vi "Read Access Key.vi"(8 "error in (no error)":errorcluster, 11 "HTTP Session in":refnum<class "Session.lvclass">) -> (0 "error out":errorcluster, 2 "Access Key":string, 3 "HTTP Session out":refnum<class "Session.lvclass">)   [LabVIEW 2015, in "NI_Azure_Core.lvlib" / "Session.lvclass"]
uses:
  Session.lvclass
  Session.lvclass/Session.ctl
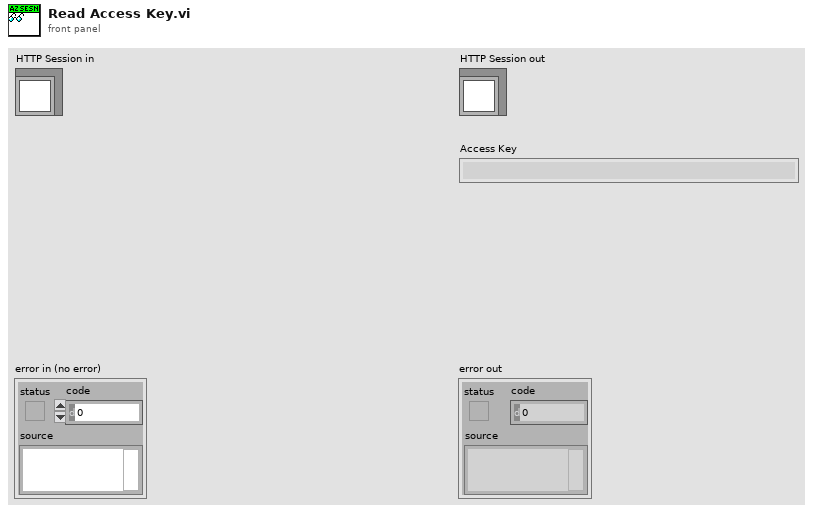
[diagram p1: front panel]
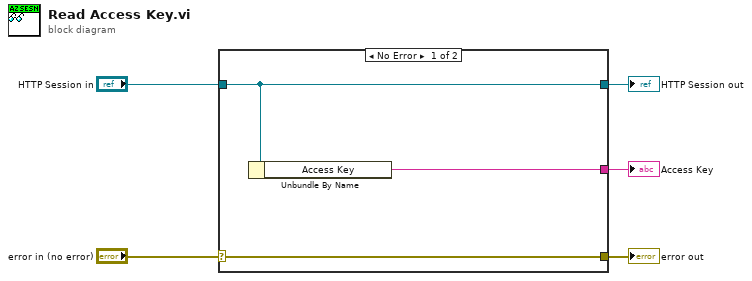
[diagram p0: block diagram]
diagram:
  n1 = case shown="No Error" "error in (no error)" {
    selector: "error in (no error)" -> [w8 w9]
    tunnel: [w8 w9] -> w4
    tunnel: [w7 w10] -> w2
    tunnel: "HTTP Session in" -> [w7 w10]
    tunnel: [w6 _] -> w1
    frame No Error {
      n2 = Unbundle By Name(w7) -> ("Access Key"=w6:string)
    }
    frame Error {
    }
  }
  "error out" <- w4
  "HTTP Session out" <- w2
  "Access Key" <- w1
